vi "Subspaces Angle (1D).vi"(10 "B":dbl[](array[numeric]), 11 "A":dbl[](array[numeric])) -> (0 "error":i32, 3 "angle":dbl)   [LabVIEW 2017, in "NI_AAL_LinAlg.lvlib"]
doc: "Computes the angle between column spaces of two matrices."
uses:
  <vilib>/Analysis/NI_AAL_LinAlg.lvlib
  <vilib>/Analysis/baseanly.llb/Unit Vector (DBL).vi
  <vilib>/Analysis/baseanly.llb/Real Dot Product.vi
  <vilib>/Analysis/NI_AALBase.lvlib
panel:
  # "Angle Between Subspaces (1D)"
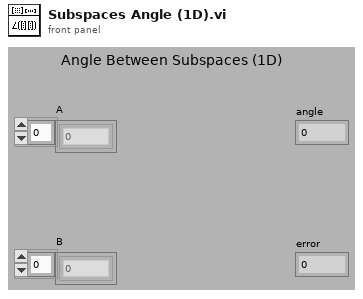
[diagram p1: front panel]
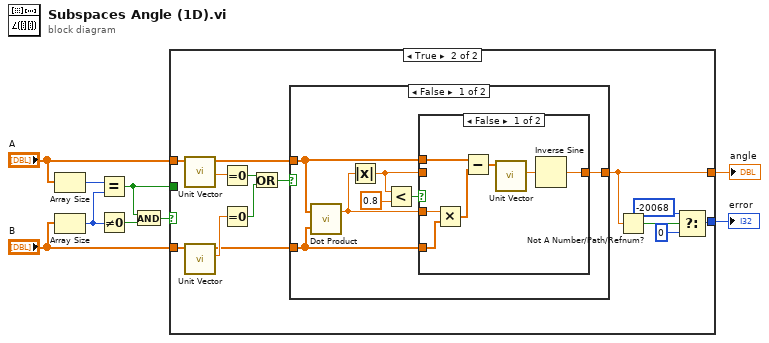
[diagram p0: block diagram]
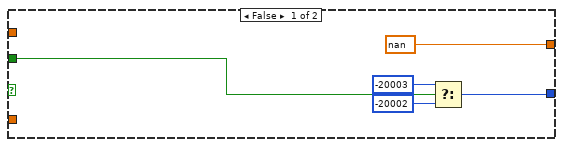
[diagram p2: hidden frame]
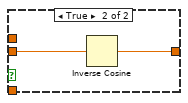
[diagram p3: hidden frame]
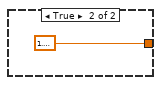
[diagram p4: hidden frame]
diagram:
  n1 = Array Size(array="A") -> (size(s)=w5:i32)
  n2 = Array Size(array="B") -> (size(s)=w4:i32)
  n3 = Equal?(x=w5, y=w4) -> (x = y?=w1:bool)
  n4 = Not Equal To 0?(x=w4) -> (x != 0?=w2:bool)
  n5 = And(x=w1, y=w2) -> (x .and. y?=w3:bool)
  n6 = case shown="True" w3 {
    tunnel: "A" -> [_ w15]
    tunnel: "B" -> [_ w28]
    tunnel: [nan w20] -> w9
    tunnel: [w13 w18] -> w8
    tunnel: w1 -> [w12 _]
    frame False {
      n7 = Select(t=-20003, s=w12, f=-20002) -> (s? t:f=w13:i32)
    }
    frame True {
      n8 = call-poly <vilib>:"Unit Vector.vi"("Input Vector"=w15) -> ("norm"=w27:dbl, "Unit Vector"=w21:dbl[])  [unwired: 2 in, 7 out]
      n9 = call-poly <vilib>:"Unit Vector.vi"("Input Vector"=w28) -> ("norm"=w26:dbl, "Unit Vector"=w22:dbl[])  [unwired: 2 in, 7 out]
      n10 = Equal To 0?(x=w27) -> (x = 0?=w25:bool)
      n11 = Equal To 0?(x=w26) -> (x = 0?=w24:bool)
      n12 = Or(x=w25, y=w24) -> (x .or. y?=w23:bool)
      n13 = case shown="False" w23 {
        tunnel: w22 -> [w34 _]
        tunnel: w21 -> [w33 _]
        tunnel: [w32 1.5707963267948966] -> w20
        frame False {
          n14 = call-poly <vilib>:"Dot Product.vi"("Y Vector"=w34, "X Vector"=w33) -> ("X * Y"=w31:dbl)  [unwired: 1 out]
          n15 = Absolute Value(x=w31) -> (abs(x)=w30:dbl)
          n16 = Less?(x=w30, y=0.8 ("threshold")) -> (x < y?=w35:bool)
          n17 = case shown="False" w35 {
            tunnel: w31 -> [w41 _]
            tunnel: w34 -> [w42 _]
            tunnel: w33 -> [w40 _]
            tunnel: [w37 w44] -> w32
            tunnel: w30 -> [_ w43]
            frame False {
              n18 = Multiply(x=w41, y=w42) -> (x*y=w39:dbl[])
              n19 = Subtract(x=w40, y=w39) -> (x-y=w38:dbl[])
              n20 = call-poly <vilib>:"Unit Vector.vi"("Input Vector"=w38) -> ("norm"=w36:dbl)  [unwired: 2 in, 8 out]
              n21 = Inverse Sine(1:w36) -> (0:w37:dbl)
            }
            frame True {
              n22 = Inverse Cosine(1:w43) -> (0:w44:dbl)
            }
          }
        }
        frame True {
        }
      }
      n23 = Not A Number/Path/Refnum?(number/path/refnum=w20) -> (NaN/Path/Refnum?=w19:bool)
      n24 = Select(t=-20068, s=w19, f=0) -> (s? t:f=w18:i32)
    }
  }
  "angle" <- w9
  "error" <- w8
